vi "Cannon Auto STOW.vi"(1 "Cannon Info In":T2) -> (0 "Cannon Info Out?":T2)   [LabVIEW 2013]
uses:
  <vilib>/Rock Robotics/WPI/Solenoid/WPI_SolenoidValue.ctl
  <vilib>/Rock Robotics/WPI/Relay/WPI_RelayValue.ctl
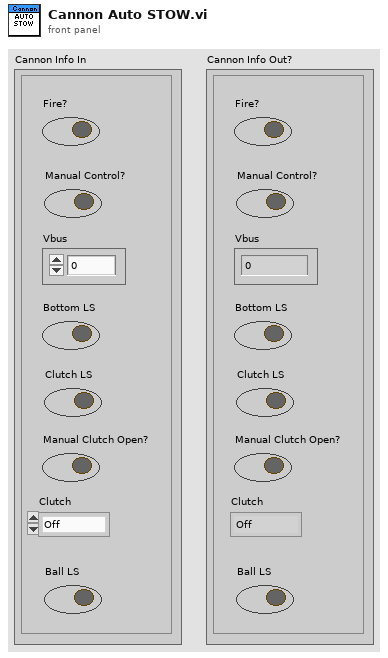
[diagram p1: front panel]
types:
  T1 = typedef "WPI_SolenoidValue.ctl" = enum16{"Off", "On", "Forward", "Reverse"}
  T2 = cluster{"Fire?":bool, "Manual Control?":bool, "Vbus":dbl, "Bottom LS":bool, "Clutch LS ":bool, "Manual Clutch Open?":bool, "Clutch":T1, "Ball LS":bool}
  T3 = typedef "WPI_RelayValue.ctl" = enum16{"Off", "On", "Forward", "Reverse"}
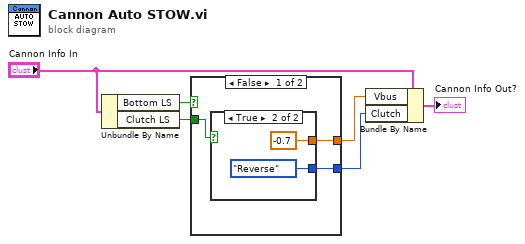
[diagram p0: block diagram]
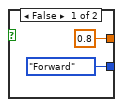
[diagram p2: hidden frame]
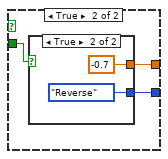
[diagram p3: hidden frame]
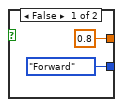
[diagram p4: hidden frame]
diagram:
  n1 = Unbundle By Name("Cannon Info In") -> ("Bottom LS"=w2:bool, "Clutch LS"=w1:bool)
  n2 = case shown="False" w2 {
    tunnel: [w8 w16] -> w3
    tunnel: [w9 w15] -> w4
    tunnel: w1 -> [w7 w14]
    frame False {
      n3 = case shown="True" w7 {
        tunnel: [0.8 -0.7] -> w8
        tunnel: [WPI_RelayValue."Forward" ("Clutch") WPI_RelayValue."Reverse" ("Clutch")] -> w9
        frame False {
        }
        frame True {
        }
      }
    }
    frame True {
      n4 = case shown="True" w14 {
        tunnel: [0.8 -0.7] -> w16
        tunnel: [WPI_RelayValue."Forward" ("Clutch") WPI_RelayValue."Reverse" ("Clutch")] -> w15
        frame False {
        }
        frame True {
        }
      }
    }
  }
  n5 = Bundle By Name(cluster="Cannon Info In", "Vbus"=w3, "Clutch"=w4) -> (→"Cannon Info Out?":T2)
